vi "getSelectedObjects.vi"(8 "error in (no error)":errorcluster, 11 "BlockDiagram in":refnum<class "BlockDiagram.lvclass">) -> (0 "error out":errorcluster, 2 "selectedGObjects":refnum<class "GObject.lvclass">[](array[class]), 3 "BlockDiagram out":refnum<class "BlockDiagram.lvclass">)   [LabVIEW 2023, in "TLC_Scripto.lvlib" / "BlockDiagram.lvclass"]
uses:
  BlockDiagram.lvclass
  GObject/GObject.lvclass
  Read GObjects.vi
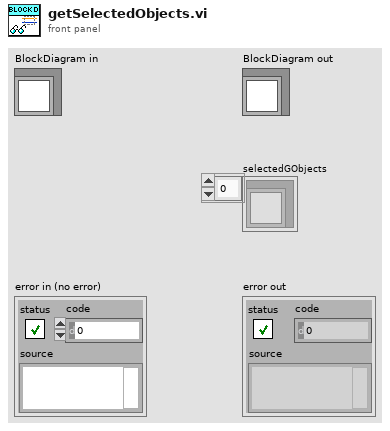
[diagram p1: front panel]
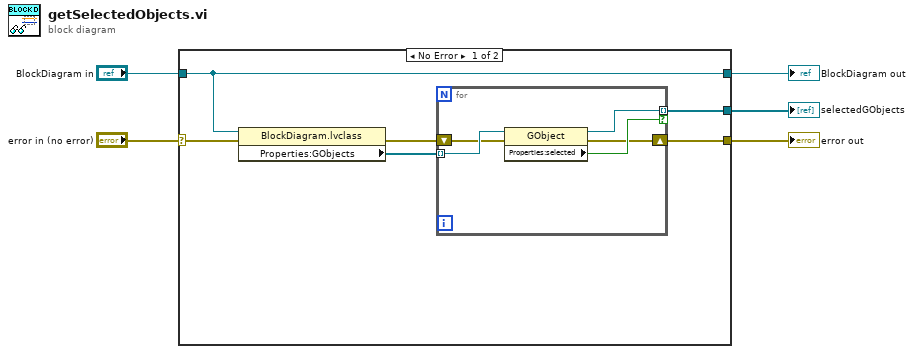
[diagram p0: block diagram]
diagram:
  n1 = case shown="No Error" "error in (no error)" {
    selector: "error in (no error)" -> [w7 w18]
    tunnel: [w8 w18] -> w4
    tunnel: [w11 w17] -> w2
    tunnel: "BlockDiagram in" -> [w11 w17]
    tunnel: [w9 _] -> w1
    frame No Error {
      n2 = property class="BlockDiagram.lvclass"(reference=w11, error in=w7) -> (error out=w6:errorcluster, "Properties:GObjects"=w10:refnum<class "GObject.lvclass">[])  [unwired: 1 out]
      n3 = for {
        tunnel: w10 -> [w16] mode=indexing
        tunnel: [w15] -> w9 mode=indexing if=w14
        shift-right: [w12] -> w8
        shift-left: w6 -> [w13]
        n4 = property class="GObject"(reference=w16, error in=w13) -> (reference out=w15:refnum<class "GObject.lvclass">, error out=w12:errorcluster, "Properties:selected"=w14:bool)
      }
    }
    frame Error {
    }
  }
  "error out" <- w4
  "BlockDiagram out" <- w2
  "selectedGObjects" <- w1
